vi "Send Next.vi"(7 "command":T1, 8 "error in (no error)":errorcluster, 9 "Plugin ID":i32, 10 "Dispatcher Interface":refnum<class "Dispatcher Interface.lvclass">, 11 "Transfer Group in":refnum<class "Transfer Group.lvclass">) -> (0 "error out":errorcluster, 3 "Transfer Group out":refnum<class "Transfer Group.lvclass">)   [LabVIEW 2017, in "DSF Core.lvlib" / "Transfer Group.lvclass"]
uses:
  Transfer Group.lvclass
  Interfaces/Dispatcher/Dispatcher Interface.lvclass
  C:/Git/DSF/Data Sharing Framework/Source/Core/Engine/Classes/Interfaces/Interface/Interface.lvclass
  Interfaces/Dispatcher/Command.ctl
  Transfer Group.lvclass/Transfer Group.ctl
  Timing/Timing.lvclass/Timing.ctl
  Interfaces/Interface/Interface.lvclass/Interface.ctl
  Interfaces/Dispatcher/Send Dispatcher Command.vi
  Interfaces/Dispatcher/Write.vi
  Interfaces/Dispatcher/Write Dispatcher Command.vi
  Interfaces/Interface/Send Command.vi
  Interfaces/Interface/Write RT FIFO.vi
  Interfaces/Dispatcher/Class Name.vi
  VIs/VI Name.vi
  Interfaces/Interface/Errors.vi
  Interfaces/Dispatcher/Command Timeout.vi
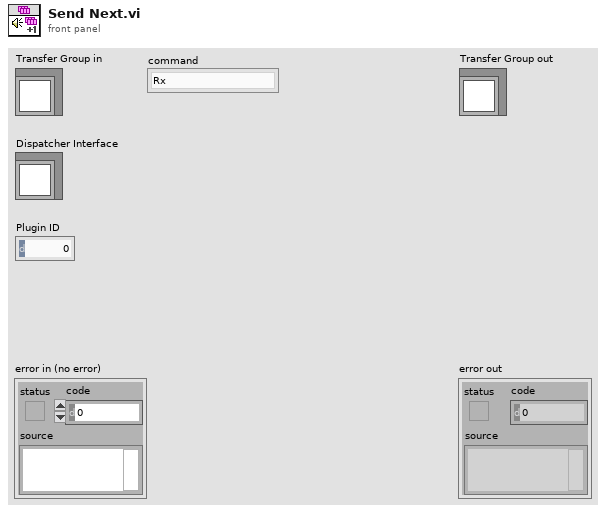
[diagram p1: front panel]
types:
  T1 = typedef "DSF Core.lvlib/Dispatcher Interface.lvclass/Command.ctl" = enum8{"Rx", "Tx", "Set Inline Buffer", "Shutdown"}
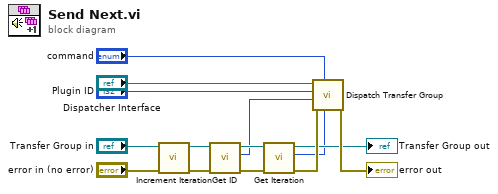
[diagram p0: block diagram]
diagram:
  n1 = call "Increment Iteration.vi"("error in (no error)"="error in (no error)", "Transfer Group in"="Transfer Group in") -> ("error out"=w11:errorcluster, "Transfer Group out"=w13:refnum<class "Transfer Group.lvclass">)  [unwired: 8 in]
  n2 = call "Get ID.vi"("Transfer Group in"=w13) -> ("id"=w10:i32, "Transfer Group out"=w12:refnum<class "Transfer Group.lvclass">)  [unwired: 9 in]
  n3 = call "Get Iteration.vi"("error in (no error)"=w11, "Transfer Group in"=w12) -> ("error out"=w9:errorcluster, "iteration"=w3:u64, "Transfer Group out"=→"Transfer Group out":refnum<class "Transfer Group.lvclass">)  [unwired: 7 in]
  n4 = call "Dispatch Transfer Group.vi"("Iteration"=w3, "command"="command", "error in (no error)"=w9, "Transfer Group ID"=w10, "Plugin ID"="Plugin ID", "Dispatcher Interface in"="Dispatcher Interface") -> ("error out"=→"error out":errorcluster)  [unwired: 4 in, 1 out]
